vi "AlliGator Color Map Phasor in Original Image v3.vi"(7 "Image Color Scale Information":T2, 8 "Error In":errorcluster, 10 "Source Image Display":T1, 11 "AlliGator IV DVR in":refnum<data-value>) -> (0 "Error Out":errorcluster, 1 "# Overlay Pixels":i32, 2 "Source Image Display":T1, 3 "AlliGator IV DVR out":refnum<data-value>)   [LabVIEW 2021, in "AlliGator Phasor Plot Color Map.lvlib"]
doc: "Overlays a color-coded map on the Source Image based on the location of each pixel's phasor with respect to the user-defined <B>Color Map</B>, a polygon in the Phasor Plot, with one color associated with each vertex."
uses:
  AlliGator Phasor Plot Color Map.lvlib
  <vilib>/vision/Image Controls.llb/IMAQ Image.ctl
  Internal Variables/AlliGator Internal Variables v2.ctl
  Internal Variables/AlliGator Gate Image Set.ctl
  Files/AlliGator FLI Dataset Type.ctl
  Files/AlliGator Data Series Type.ctl
  Dual-Channel Datasets/AlliGator Dataset Channel.ctl
  Settings/AlliGator Gate Arithmetic.ctl
  Source Image/AlliGator Displayed Image.ctl
  Image/Named ROI Description.ctl
  Phasor Graph/AlliGator Decay Metadata v3.ctl
  Decay Analysis/Decay Preprocessing/AlliGator Decay Background Subtraction Info.ctl
  Decay Analysis/Decay Preprocessing/AlliGator Baseline Subtraction Method.ctl
  Graphs/XY Graph/XY Graph Plot Shift Parameters.ctl
  Graphs/XY Graph/XY Graph Plot Shift Method.ctl
  Decay Analysis/Decay Preprocessing/AlliGator Decay Extrapolation Parameters.ctl
  Phasor/Calibration Phasor (m, phi).ctl
  Phasor/Phasor Reference Series.ctl
  Phasor/Phasor Calibration Map v2.ctl
  Phasor/Phasor (g, s).ctl
  Phasor Graph/AlliGator Raw Phasor Plot Data v4.ctl
  Phasor/Phasor Standard Deviation Options.ctl
  Phasor Plot/AlliGator Phasor Multi-Harmonic Data.ctl
  Phasor/Phasor Harmonic Data.ctl
  Decay Fit Parameter Map/AlliGator Decay Fit Options & Parameters v2.ctl
  Fits/IRF(X)PSED/Decay Fit Options v2.ctl
  Fits/Decay Convolution/Decay Model.ctl
  Fits/Residual Type.ctl
  Fits/IRF(X)PSED/Fit Weights Type.ctl
  Fits/Non-linear Fitting Method v2.ctl
  Fits/Fit Calculation Method.ctl
  Fits/Non-linear Fitting Algorithm.ctl
  Decay Analysis/Decay Fit/AlliGator Decay Fit Parameter Constraints 2.ctl
  Fits/IRF(X)PSED/Decay Fit Parameters In List.ctl
  Fits/IRF(X)PSED/MLE Baseline Offset Type.ctl
  Decay Analysis/Decay Preprocessing/AlliGator Decay Preprocessing Parameters.ctl
  Fits/IRF(X)PSED/Decay Fit Parameters & Derived Quantities List v2.ctl
  Decay Fit Parameter Map/AlliGator Parameter Maps Data.ctl
  Image/Image Color Scale Information.ctl
  Settings/AlliGator Settings List.ctl
  Palette/Image Palette Information.ctl
  Image/Image Display Palette Type.ctl
  Globals, Variables, Constants/AlliGator Variables List.ctl
  Variant/Variant to Data/Variant to Boolean.vi
  <vilib>/Analysis/geometry.llb/Point in Polygon (Scalar).vi
  Image/Image Get Pixel Color.vi
  Image/Adjust Pixel Overlay Brightness.vi
  <vilib>/vision/NI_Vision_Development_Module.lvlib
  Error/Error.lvlib
  Image/Image.lvlib
  <vilib>/Analysis/NI_AAL_Geometry.lvlib
  Settings/AlliGator Settings.lvlib
  Variant/Variant to Data/Variant to Data.lvlib
  Time/Time.lvlib
  Utilities/Utilities.lvlib
  Globals, Variables, Constants/AlliGator Globals, Variables & Constants.lvlib
  Palette/Palette.lvlib
  Phasor/Phasor.lvlib
  Decay Analysis/Decay Preprocessing/AlliGator Decay Preprocessing.lvlib
  Graphs/XY Graph/XY Graph Add-Ons.lvlib
  Phasor Graph/AlliGator Phasor Graph.lvlib
  Files/AlliGator Files.lvlib
  Phasor Plot/AlliGator Phasor Plot.lvlib
  Source Image/AlliGator Source Image.lvlib
  Internal Variables/AlliGator Internal Variables.lvlib
  Fits/Fits.lvlib
  Decay Analysis/Decay Fit/AlliGator Decay Fit.lvlib
  Decay Fit Parameter Map/AlliGator Decay Fit Parameter Map.lvlib
  Dual-Channel Datasets/AlliGator Dual-Channel Datasets.lvlib
panel:
  out "Overlay Copy (s)":dbl
  out "Overlay Erase (s)":dbl
  out "Overlay Compute (s)":dbl
  # "see the AlliGator License on the block diagram (Ctrl+E or Window:Show Block Diagram)"
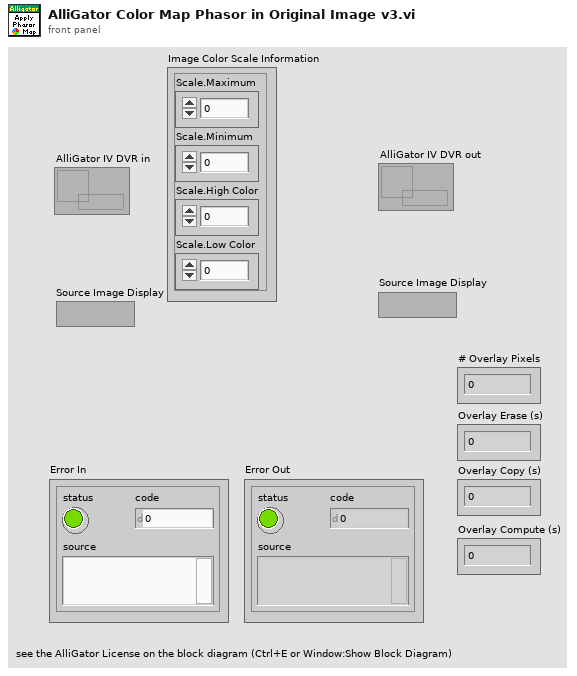
[diagram p1: front panel]
types:
  T1 = typedef "IMAQ Image.ctl" = refnum<image>
  T2 = typedef "Image.lvlib/Image Color Scale Information.ctl" = cluster{"Scale.Maximum":dbl, "Scale.Minimum":dbl, "Scale.High Color":u32, "Scale.Low Color":u32}
  T3 = typedef "AlliGator Settings.lvlib/AlliGator Settings List.ctl" = enum16{"GUI:Visible Settings Tab", "GUI:Last Run Version", "Source Image:Use Image Histogram for Contrast", "Source Image:Low Count Pixels Rejection Options", "Source Image:High Count Pixels Rejection Options", "Source Image:Use Image Brightness", "Source Image:Blend Overlay with Image Background", "Source Image:Use Fixed ROI Diameter", "Source Image:ROI Diameter", "Source Image:ROI Center Color", "Source Image:Peak Threshold", "Source Image:Intensity Threshold", "Source Image:Image Binning Options", "Source Image:Image Smoothing Options", "Source Image:Image Histogram Active", "Source Image:Invert Binary Mask", "Source Image:Hot Pixel Removal", "Source Image:Overlay Analyzed ROI Center", "Source Image:Auto-Adjust Contrast", "Source Image:Histogram Lower Percentile", "Source Image:Histogram Upper Percentile", "Source Image:Save Source Image", "Source Image:Scale Bar Options", "Source Image:Image Resolution (Pixel Size)", "Source Image:Flatfield Correction", "Source Image:Show Dead Left Columns Correction", "Source Image:Dead Left Columns Correction", "Source Image:Image Pre-Processing Operations Order", "Source Image:Overlay ROI Median", "Source Image:Median Overlay Color", "Data Information:Gate Width", "Data Information:Nanotime Gate Separation", "Data Information:Macrotime Gate Separation", "Data Information:Gate Step", "Data Information:# Gates", "Data Information:Gate Image Exposure", "Data Information:Gate Image Integration", "Data Information:Gates to Skip", "Data Information:Gates to Keep", "Data Information:Define Gates to", "Data Information:Channel Name", "Data Information:Available Channel Names", "Data Information:Channel Arithmetic", "Data Information:Background File Subtraction", "Data Information:Background File", "Data Information:Background Scaling Factor", "Data Information:Background Pile-up Correction", "Data Information:Background Pixel Well Capacity", "Data Information:Laser Period", "Data Information:SYNC Period", "Data Information:Pile-up Correction", "Data Information:Pixel Well Capacity", "Data Information:Dataset Scaling Factor", "Fluorescence Decay_Decay Pre-Processing:Reverse Gates", "Fluorescence Decay_Decay Pre-Processing:Verbose Decay Pre-Processing", "Fluorescence Decay_Decay Pre-Processing:Use Decay Pre-Processing", "Fluorescence Decay_Decay Pre-Processing:Background Subtraction", "Fluorescence Decay_Decay Pre-Processing:Background Definition Range", "Fluorescence Decay_Decay Pre-Processing:Baseline Subtraction Method", "Fluorescence Decay_Decay Pre-Processing:Decay Pre-Processing Operations Order", "Fluorescence Decay_Decay Pre-Processing:Smoothing Parameter", "Fluorescence Decay_Decay Pre-Processing:Shift Decay", "Fluorescence Decay_Decay Pre-Processing:Decay Shift Parameters", "Fluorescence Decay_Decay Pre-Processing:Fold Decay", "Fluorescence Decay_Decay Pre-Processing:# Folds", "Fluorescence Decay_Decay Pre-Processing:1-Normalize Decay", "Fluorescence Decay_Decay Pre-Processing:[0-1]-Normalize Decay", "Fluorescence Decay_Decay Pre-Processing:Smoothen Decay", "Fluorescence Decay_Decay Pre-Processing:Extrapolate Decay", "Fluorescence Decay_Decay Pre-Processing:Use Periodicity", "Fluorescence Decay_Decay Pre-Processing:Use Cursors", "Fluorescence Decay_Decay Pre-Processing:Tail Fraction", "Fluorescence Decay_Decay Pre-Processing:Head Fraction", "Fluorescence Decay_Decay Pre-Processing:Additional Points", "Fluorescence Decay_Decay Pre-Processing:Straighten Decay", "Fluorescence Decay_Decay Pre-Processing:Constant Background", "Fluorescence Decay_Decay Pre-Processing:Pixel-Normalize Decay", "Fluorescence Decay_Advanced Analysis:Extract IRF instead of Decay", "Fluorescence Decay_Advanced Analysis:IRF Extraction Options", "Fluorescence Decay_Advanced Analysis:IRF Optimization Options", "Fluorescence Decay_Advanced Analysis:Square Pulse Options", "Fluorescence Decay_Advanced Analysis:IRF Order", "Fluorescence Decay_Advanced Analysis:IRF Time Constants", "Fluorescence Decay_Advanced Analysis:Wavelet Analysis Options", "Fluorescence Decay_Advanced Analysis:Average Lifetime Options", "Fluorescence Decay_Fit Options:Fit Options", "Fluorescence Decay_Fit Options:Use Legacy Fitting Approach", "Fluorescence Decay_Fit Options:Use Data Information Laser Period", "Fluorescence Decay_Fit Parameters:Displayed Fit Parameters", "Fluorescence Decay_Fit Parameters:Fit Parameter Constraints", "Fluorescence Decay_Fit Parameters:Export Tabulated Results", "Fluorescence Decay_Fit Parameters:MLE Baseline Offset Type", "Fluorescence Decay_Fit Parameters:MLE Baseline Offset", "Fluorescence Decay_Fit Parameters:Guess Parameter Names", "Fluorescence Decay_Fit Parameters:Guess Parameter Values", "Fluorescence Decay_Fit Parameters:Guess Parameters Options", "Fluorescence Decay_Styles:Show Last Decay Only", "Fluorescence Decay_Styles:Decay Graph Color Array", "Fluorescence Decay:Decay Graph Active", "Fluorescence Decay Statistics:Min Peak Value", "Fluorescence Decay Statistics:Reject Low Decay Peak Pixels", "Fluorescence Decay Statistics:Reject High Decay Peak Pixels", "Fluorescence Decay Statistics:Max Peak Value", "Time Traces:Use File Timestamp", "Time Traces:Time Step", "Time Traces:Use Intensity Correction File", "Time Traces:Intensity Correction File", "Phasor Plot:Phasor Plot Smoothing Options", "Phasor Plot:Phasor Plot Size", "Phasor Plot:Phasor Plot Graphics Options", "Phasor Plot:Cumulative Phasor Plot", "Phasor Plot:Use Phasor Brightness", "Phasor Plot:Blend Overlay with Phasor Background", "Phasor Plot:Save Phasor Plot", "Phasor Plot:Show References", "Phasor Plot:Phasor Ratio Decay Range", "Phasor Plot:Exponential Fading", "Phasor Plot:Phasor Ratio Reference Colors", "Phasor Plot:Reference Radius", "Phasor Plot:Show Color Map Vertices", "Phasor Plot:Phasor Plot Active", "Phasor Plot:Phasor Ratio Color Map Type", "Phasor Plot:Phasor Ratio Color Map", "Phasor Plot:Phasor Ratio Display Range", "Phasor Plot:Selected Image ROI(s)", "Phasor Plot:All Image ROIs", "Phasor Plot:Selected Phasor Plot ROI(s)", "Phasor Plot:All Phasor Plot ROIs", "Phasor Plot:Phasor Ratio Color-Coded Quantity", "Phasor Plot:Store Phasor Harmonics", "Phasor Plot:Draw Reference Segment", "Phasor Plot:User-Defined Quantity", "Phasor Graph:Phasor Frequency", "Phasor Graph:Phasor Ratio Type", "Phasor Graph:Pixel-level Phasor Computation", "Phasor Graph:Save Phasor Graph", "Phasor Graph:Phasor Graph Active", "Phasor Graph:Phasor SDV Options", "Phasor Calibration:Use Backup Calibration if needed", "Phasor Graph:Define Shortest Lifetime as", "Phasor Calibration:Backup Calibration Type", "Phasor Calibration:Calibration Type", "Phasor Calibration:Calibration Lifetime", "Phasor Calibration:Calibration Map Algorithm", "Single-Exponential Phasor Locus (SEPL):Gate Parameters", "Single-Exponential Phasor Locus (SEPL):User-defined Gate", "Single-Exponential Phasor Locus (SEPL):User-defined IRF", "Single-Exponential Phasor Locus (SEPL):Phasor Parameters", "Single-Exponential Phasor Locus (SEPL):Decay & IRF Parameters", "Single-Exponential Phasor Locus (SEPL):Display Parameters", "Lifetime Analysis:Decay Analysis Parameters", "Lifetime Analysis:Lifetime Map Active", "Plugins:Python Settings", "Miscellaneous:Verbose Mode", "Miscellaneous:Beep after Script", "Miscellaneous:Saved Image File Format", "Miscellaneous:Exported Gate Image Settings", "Miscellaneous:Include Loading in Timing", "Miscellaneous:Verbose Settings Mode", "Miscellaneous:Histogram Options", "Miscellaneous:Beep on Error", "Miscellaneous:# Logical Processors Used", "Miscellaneous:ROI Description Max Characters", "Miscellaneous:Verbose Error Mode", "Miscellaneous:Transparent Mask Color"}
  T4 = typedef "Palette.lvlib/Image Palette Information.ctl" = cluster{"Palette Name [# Colors,int?,inv?]":string, "Palette Type":T5, "Palette Colors":u32[], "Interpolate?":bool}
  T5 = typedef "Image.lvlib/Image Display Palette Type.ctl" = u32
  T6 = typedef "AlliGator Globals, Variables & Constants.lvlib/AlliGator Variables List.ctl" = enum16{"---- GUI ----", "GUI:Initialization Status", "GUI:State Indicators Refnum", "GUI:Original AlliGator Menu Items", "GUI:Current Action Loop State", "GUI:Script in progress", "GUI:Playback", "GUI:Loop Playback", "GUI:Search ROI Used", "GUI:Search ROI", "Decay Graph Max Legend Size", "Intensity Graph Max Legend Size", "Decay Statistics Graph Max Legend Size", "Phasor Graph Max Legend Size", "Phasor Ratio Graph Max Legend Size", "Lifetime Graph Max Legend Size", "---- Files ----", "Files:Export Dataset Frames as Individual Files", "Files:Show Batch Export Help Balloons", "Files:Frames in Dataset", "Files:ptu File Frame Start Indices", "Files:Current Frame in Dataset", "Files:Current Frame Timestamp", "Files:Dataset Loaded", "Files:Dataset Metadata", "Files:Dataset Channel", "Files:Dataset Data Description", "Files:Background Dataset Metadata", "Files:Background Dataset Channel", "Files:Background Dataset Data Description", "Files:Background File Subtraction", "Files:Background File Path", "Files:Background File Pile-up Correction", "Files:Background File Pixel Well Capacity", "Files:Background File Scaling Factor", "Files:Current Dataset Load Settings", "Files:Dataset Path", "Files:ICCD-specific Information", "Files:Macrotime Gate Separation", "------ Python Plugins ------", "Python Plugins:Information", "Python Plugins:Python Session", "Python Plugins:Valid Python Session?", "---- Source Image ----", "Source Image:ROIs", "Source Image:Current ROI", "Source Image:ROI Event Refnum", "X_Source Image Display Range", "X_Source Image Palette Information", "X_Type of Displayed Image", "X_Time Gate Slider", "Source Image:Palette List", "Source Image:Scale", "Source Image:ROI Overlay Color", "Source Image:Overlay to Erase", "Source Image:Is Displayed Image Accumulated", "Source Image:White Light Image Modified", "Source Image:Mask Image Modified", "---- Image Profile Window ----", "Image Profile:Window Event Refnum", "Image Profile:IntensityType", "Image Profile:Intensity Average Type", "Image Profile:Intensity-weighted SDV", "Image Profile:Box Profile Type", "Image Profile:Window Open", "Image Profile:Plotted Fit Parameter", "------ Phasor Graph -------", "Phasor Graph:Show Line", "---- Phasor Plot ---", "Phasor Plot:Parameters Changed", "Phasor Plot:FLI Dataset Modified since last Calculation", "Phasor Harmonics Data", "Selected Phasor Harmonics", "Phasor Harmonic Manager Event Refnum", "Phasor Plot:ROIs", "Phasor Plot:Current ROI", "Phasor Plot:ROI Event Refnum", "Phasor Plot:Image Reference Points", "Phasor Plot:Computed", "Phasor Plot:Palette Information", "Phasor Plot:Palette List", "Phasor Plot:Phasor Ratio Palette Information", "Phasor Plot:Phasor Ratio Palette List", "Phasor Plot:Image Scale", "Phasor Plot:Image Overlay to Erase", "Phasor Plot:Image Elements to Update", "Phasor Plot:Current Calculation Parameters", "Phasor Plot:Current Calibration Options", "Phasor Plot:Reset Cumulated Phasor Plot", "Phasor Plot:Reference 1", "Phasor Plot:Lifetime Reference 1", "Phasor Plot:Reference 1 Frequency", "Phasor Plot:Reference 2", "Phasor Plot:Lifetime Reference 2", "Phasor Plot:Reference 2 Frequency", "---- Decay Analysis ----", "Number of Selected Decays to Fit", "LS Fit Results", "LAR Fit Results", "BS Fit Results", "Last Decay Max - Min", "Best Fit Parameters", "Best Fit Parameter Names", "Actual Size X", "Actual Size Y", "Binning X", "Binning Y", "Actual # Gates", "Dataset Number", "Gates to...", "Gates Skipped", "Gates to keep", "Gate Step", "Gate Separation", "Reversed Gates", "Pile-up Correction", "Pixel Well Capacity", "Background Subtracted", "Background Subtraction Method", "Background Definition Range", "Background File (deprecated)", "Number of Dataset Accumulated", "Array of Accumulated Dataset Paths", "Do Averaged Datasets", "Destination File Path", "Process Plot Target", "Use 1/D as Phasor Frequency", "---- Decay Fit Parameter Map -----", "Decay Fit Parameter Map:Palette Information", "Decay Fit Parameter Map:Palette List", "---- Parameter Map ----", "Parameter Map:Palette Information", "Parameter Map:Palette List", "------- Local Decay Window ---------", "Local Decay Graph Window:Event Refnum", "Local Decay Graph Window:Use normalized IRF for convolution", "----- Miscellaneous ----", "Misc:Skippable Dialog Windows Status"}
  T7 = typedef "AlliGator Internal Variables.lvlib/AlliGator Internal Variables v2.ctl" = cluster{"Displayed Image":T1, "White Light Image":T1, "Mask Image":T1, "ROI Mask Image":T1, "Current Dataset Images 1":T8, "Background Dataset Images 1":T8, "Current Dataset Images 2":T8, "Background Dataset Images 2":T8, "Current Dataset Arithmetic Images":T8, "Accumulated Dataset Images 1":T8, "Accumulated Dataset Images 2":T8, "Accumulated Dataset Arithmetic Images":T8, "Phasor Plot Image":T1, "Decay Fit Parameter Map Image":T1, "Parameter Map Image":T1, "Single Data Point Path":path, "White Light Image Path":path, "Mask Image Path":path, "Time-Series Folder":path, "[Time-Series Paths]":path[], "Current Dataset":i32, "Single Dataset Type":T9, "Current Folder":string, "AlliGator Data Series Type":T10, "# Datasets":i32, "Dual-Channel Dataset":bool, "Selected Channel Name":string, "Dataset Channel":T11, "Channel Arithmetic":T12, "Dual-Channel Background Dataset":bool, "Background Channel":T11, "Dual-Channel Accumulated Dataset":bool, "Start Time":dbl, "[Time-Series Timestamps]":dbl[], "[Intensity Corrections]":dbl[], "Time Series Script":bool, "Type of Displayed Image":T13, "Gate Image Slide":u16, "# Gates":i32, "ROIs":T14[], "ROI Decay":cluster{"t Array":dbl[], "I Array":dbl[]}, "Valid Decay":bool, "Decay  Metadata":T16, "Reference Decay Plot Name":string, "Reference Decay":cluster{"t Array":dbl[], "I Array":dbl[]}, "Decay Shift Plot":cluster{"Time Stamps":dbl[], "Decay Shifts":dbl[]}, "[Decays Max Values]":sgl[], "[Decays Min Values]":sgl[], "Calibration Phasor":T22, "Calibration Phasor Series":T23, "Phasor Calibration Map":T24, "Calibration Map MD5 Digest":string, "Last Raw Phasor":T25, "Last Calibrated Phasor":T25, "Last Calibrated Phasor SDV":T25, "Phasor Graph:Phasor Plot":cluster{"g Array":dbl[], "s Array":dbl[]}, "Phasor Graph:Phasor SDV Plot":cluster{"g Array":dbl[], "s Array":dbl[]}, "[Phasor Graph:Raw Phasor Plots]":T26[], "Phasor Plot locked to Ref 1":i32, "[Phasor Plot(s) locked to Ref 1]":i32[], "[Phasor Plot(s) locked to Ref 2]":i32[], "[Pixel Phasors]":T25[], "[[Sum Image]]":dbl[][], "[[CSG Phasors]]":csg[][], "[[Valid Pixel?]]":bool[][], "I/m/phi Dataset":cluster{"I/m/phi Dataset?":bool, "Base Frequency":dbl[unit], "Harmonic Orders":u8[]}, "Multi Phasor Plot Data":T28, "Decay Fit Options & Parameters":T30, "Fit Options: Decay Preprocessing Parameters":T41, "Fit Options: Reference Decay":cluster{"t Array":dbl[], "I Array":dbl[]}, "Is Full Image Parameters Map":bool, "Is Single-Pixels Parameters Map":bool, "NLSF Parameters Map X Resolution":i32, "NLSF Parameters Map Y Resolution":i32, "[Single Decay Fit Parameters]":dbl[], "Fit Model":T32, "[[Multiple Decays Fit Parameters]]":dbl[][], "[[Multiple Decays Fit Parameter SDVs]]":dbl[][], "[[IRFs]]":dbl[][], "IRF Array Time Axis":dbl[], "Decay Array Time Axis":dbl[], "[Decay Fit Parameter Names]":T42[], "[[Phasor Ratios]]":dbl[][], "[[Average Lifetimes]]":dbl[][], "Amplitude Weighted Average Lifetime":bool, "[Decay Sum]":dbl[], "[Map Set Names]":string[], "[Parameter Maps]":T43[], "[[User-defined Quantities]]":dbl[][], "User-defined Quantity":string}
  T8 = typedef "AlliGator Internal Variables.lvlib/AlliGator Gate Image Set.ctl" = cluster{"SGL Image Max":T1, "SGL Image Sum":T1, "SGL Gate Images":T1[], "SGL Image Min":T1}
  T9 = typedef "AlliGator Files.lvlib/AlliGator FLI Dataset Type.ctl" = enum16{"HDF5 FLI Dataset", "Gate Image Folder", ".sdt FLI Dataset (Becker & Hickl)", ".ptu FLI Dataset (PicoQuant)", "SS1 FLI Dataset", "SS2 FLI Dataset", "I/m/phi Dataset", ".bin FLI Dataset (PicoQuant Binned)", ".bin FLI Dataset (Piccolo Binned)"}
  T10 = typedef "AlliGator Files.lvlib/AlliGator Data Series Type.ctl" = enum16{"Not a Supported Series", "Gate Images Folder Series", "SwissSPAD 2 Dataset Series", "B&H FLI Dataset Series", "PicoQuant PTU FLI Dataset Series", "PicoQuant BIN FLI Dataset Series", "Piccolo hist BIN FLI Dataset Series", "HDF5 FLI Dataset Series"}
  T11 = typedef "AlliGator Dual-Channel Datasets.lvlib/AlliGator Dataset Channel.ctl" = enum16{"G2", "INT"}
  T12 = typedef "AlliGator Settings.lvlib/AlliGator Gate Arithmetic.ctl" = enum16{"None", "INT-G2", "G2/INT*<INT>", "(1 - G2/INT)*<INT>"}
  T13 = typedef "AlliGator Source Image.lvlib/AlliGator Displayed Image.ctl" = enum16{"Single Gate", "Sum of All Gates", "Max of All Gates", "Min of All Gates", "-", "White Ligth Image", "Mask Image"}
  T14 = typedef "Image.lvlib/Named ROI Description.ctl" = cluster{"ROI Descriptor":T15, "ROI Name":string, "Overlay Color":u32}
  T15 = typedef "ROI Descriptor" = cluster{"Global Rectangle":i32[], "Contours":cluster{"ID":enum32{"External", "Internal"}, "Type":u32, "Coordinates":i32[]}[]}
  T16 = typedef "AlliGator Phasor Graph.lvlib/AlliGator Decay Metadata v3.ctl" = cluster{"ROI Descriptor":T15, "ROI Center":cluster{"X":i32, "Y":i32}, "Decay Background Subtraction Info":T17, "Decay Reverted":bool, "Decay Smoothened":bool, "Decay Straightened":bool, "Fitted Tau (Decay Straightening)":dbl, "Decay Shift Parameters":T19, "Decay Shifted":bool, "Decay Extrapolated":bool, "Decay Extrapolation Parameters":T21, "Decay Normalized":bool, "Fold Decay":bool, "# Folds":u32}
  T17 = typedef "AlliGator Decay Preprocessing.lvlib/AlliGator Decay Background Subtraction Info.ctl" = cluster{"Laser Period":dbl[unit], "Gate Duration":dbl[unit], "Baseline Subtraction Method":T18, "Background Definition Range":cluster{"Min Gate":dbl[unit], "Max Gate":dbl[unit]}, "Total Intensity w/o Bkgd Subtraction":dbl, "Bkgd-subtracted Intensity (exp)":dbl, "# Data Points":i32, "Background/Gate":dbl, "Fitted Lifetime":dbl[unit], "Bkgd-subtracted Intensity (theo)":dbl}
  T18 = typedef "AlliGator Decay Preprocessing.lvlib/AlliGator Baseline Subtraction Method.ctl" = enum16{"Mean", "Min", "Square Gated Single-Exponential", "File", "Constant"}
  T19 = typedef "XY Graph Add-Ons.lvlib/XY Graph Plot Shift Parameters.ctl" = cluster{"Type":T20, "Shift":dbl[unit], "Threshold":dbl, "Rotate":bool}
  T20 = typedef "XY Graph Add-Ons.lvlib/XY Graph Plot Shift Method.ctl" = enum16{"Default", "CFD", "Threshold", "Cross-Correlation"}
  T21 = typedef "AlliGator Decay Preprocessing.lvlib/AlliGator Decay Extrapolation Parameters.ctl" = cluster{"Additional Points":u32, "Head Fraction":dbl, "Fitted Tau":dbl, "Use Periodicity":bool, "Use Cursors":bool, "Tail Fraction":dbl}
  T22 = typedef "Phasor.lvlib/Calibration Phasor (m, phi).ctl" = cluster{"m":dbl, "phi":dbl, "Phasor Frequency":dbl[unit], "Reference Lifetime":dbl[unit]}
  T23 = typedef "Phasor.lvlib/Phasor Reference Series.ctl" = cluster{"m Array":dbl[], "phi Array":dbl[], "Phasor Frequency":dbl[unit], "Calibration Lifetime":dbl[unit]}
  T24 = typedef "Phasor.lvlib/Phasor Calibration Map v2.ctl" = cluster{"Phasor Frequency":dbl[unit], "Calibration Lifetime":dbl[unit], "ROI Centers":cluster{"X":i32, "Y":i32}[], "ROI Descriptors":T15[], "Map Resolution X":i32, "Map Resolution Y":i32, "z Array":cdb[]}
  T25 = typedef "Phasor.lvlib/Phasor (g, s).ctl" = cluster{"g":dbl, "s":dbl}
  T26 = typedef "AlliGator Phasor Graph.lvlib/AlliGator Raw Phasor Plot Data v4.ctl" = cluster{"Phasor Plot Name":string, "Raw Phasor Plot":T25[], "Phasor Frequency":dbl[unit], "[Decay Metadata]":T16[], "Raw Phasor Plot SDV":T25[], "Phasor SDV Options":T27, "[Calibration Phasor]":T22[]}
  T27 = typedef "Phasor.lvlib/Phasor Standard Deviation Options.ctl" = cluster{"Compute Estimated SDV":bool, "# Replicas":u32, "Use Estimated Average Phasor":bool}
  T28 = typedef "AlliGator Phasor Plot.lvlib/AlliGator Phasor Multi-Harmonic Data.ctl" = cluster{"Base Frequency":dbl[unit], "# Harmonics":u8, "Harmonic Orders":u8[], "Phasor Plot Settings Checksum":u64, "Phasor Harmonic Data Array":T29[]}
  T29 = typedef "Phasor.lvlib/Phasor Harmonic Data.ctl" = cluster{"Phasor Harmonic Name":string, "Phasor Plot Settings Checksum":u64, "Phasor Frequency":dbl[unit], "Base Frequency":dbl[unit], "Harmonic Order":u8, "Phasor Plot Parameters":string, "Phasor Array [[CSG]]":csg[][], "Dataset File Path":path}
  T30 = typedef "AlliGator Decay Fit Parameter Map.lvlib/AlliGator Decay Fit Options & Parameters v2.ctl" = cluster{"SYNC Period":dbl[unit], "Fit Options":T31, "Fit Parameter Constraints":T38[], "MLE Baseline Offset":dbl, "MLE Baseline Offset Type":T40}
  T31 = typedef "Fits.lvlib/Decay Fit Options v2.ctl" = cluster{"Show Fit Residuals":bool, "Fit Model":T32, "Residual Type":T33, "Max Decay Percentile":dbl, "Min Decay Percentile":dbl, "Show Full Decay":bool, "Weights":T34, "Fitting Method":T35, "Compute Parameter Uncertainties":bool, "Periodic Boundaries":bool, "Model Calculation":T36, "Period":dbl[unit], "Termination Criteria":cluster{"Max Iterations":i32, "Max Function Calls":i32, "Max Time":dbl[unit], "Function Tolerance":dbl, "Parameter Tolerance":dbl, "Gradient Tolerance":dbl, "Min Lambda":dbl, "Max Lambda":dbl, "Initial Tick Count":u32}, "Offset Resolution":dbl[unit], "Use Local IRF":bool, "Fitting Algorithm":T37}
  T32 = typedef "Fits.lvlib/Decay Model.ctl" = enum16{"1-Exponential", "2-Exponentials"}
  T33 = typedef "Fits.lvlib/Residual Type.ctl" = enum16{"Standard", "Normalized", "Reduced"}
  T34 = typedef "Fits.lvlib/Fit Weights Type.ctl" = enum16{"Unweighted", "1/Variance", "Best of All"}
  T35 = typedef "Fits.lvlib/Non-linear Fitting Method v2.ctl" = enum16{"Least Square", "Least Absolute Residual", "Bisquare", "MLE", "-", "Best of All"}
  T36 = typedef "Fits.lvlib/Fit Calculation Method.ctl" = enum16{"Simulation", "Convolution", "Integration"}
  T37 = typedef "Fits.lvlib/Non-linear Fitting Algorithm.ctl" = enum16{"Levenberg-Marquardt", "Trust-Region Dogleg"}
  T38 = typedef "AlliGator Decay Fit.lvlib/AlliGator Decay Fit Parameter Constraints 2.ctl" = cluster{"Fit Parameter":T39, "Min Value":dbl, "Max Value":dbl, "Global":bool, "Used":bool}
  T39 = typedef "Fits.lvlib/Decay Fit Parameters In List.ctl" = enum16{"Offset", "Baseline", "A_1", "tau_1", "A_2", "tau_2"}
  T40 = typedef "Fits.lvlib/MLE Baseline Offset Type.ctl" = enum32{"Absolute", "Percentage"}
  T41 = typedef "AlliGator Decay Preprocessing.lvlib/AlliGator Decay Preprocessing Parameters.ctl" = cluster{"Background Subtraction":bool, "Straighten Decay":bool, "Reverse Gates":bool, "1-Normalized Decay":bool, "Smoothen Decay":bool, "Smoothing Parameter":dbl, "Shift Decay":bool, "Decay Shift Parameters":T19, "Extrapolate Decay":bool, "Additional Points":u32, "Head Fraction":dbl, "Pixel-Normalize Decay":bool, "Use Periodicity":bool, "Use Cursors":bool, "Tail Fraction":dbl, "Use Decay Pre-Processing":bool, "Fold Decay":bool, "# Folds":u32, "[0-1]-Normalized Decay":bool}
  T42 = typedef "Fits.lvlib/Decay Fit Parameters & Derived Quantities List v2.ctl" = enum16{"Offset", "Baseline", "A_1", "tau_1", "A_2", "tau_2", "<tau>_a", "f1_a", "f2_a", "<tau>_i", "f1_i", "f2_i", "-", "R^2", "Chi^2"}
  T43 = typedef "AlliGator Decay Fit Parameter Map.lvlib/AlliGator Parameter Maps Data.ctl" = cluster{"Map Set Name":string, "[Parameter Names]":string[], "[[Parameters]]":dbl[][], "[[Parameter SDVs]]":dbl[][], "Decay Array Time Axis":dbl[], "[[IRFs]]":dbl[][], "IRF Array Time Axis":dbl[]}
  T44 = cluster{"Red (or Hue) value":u8, "Green (or Sat) value":u8, "Blue (or Light or Val) value":u8}[]
  T45 = typedef "NI_AAL_Geometry.lvlib/Point in Polygon Position.ctl" = u16
  T46 = cluster{"Red (or Hue) value":u8, "Green (or Sat) value":u8, "Blue (or Light or Val) value":u8}
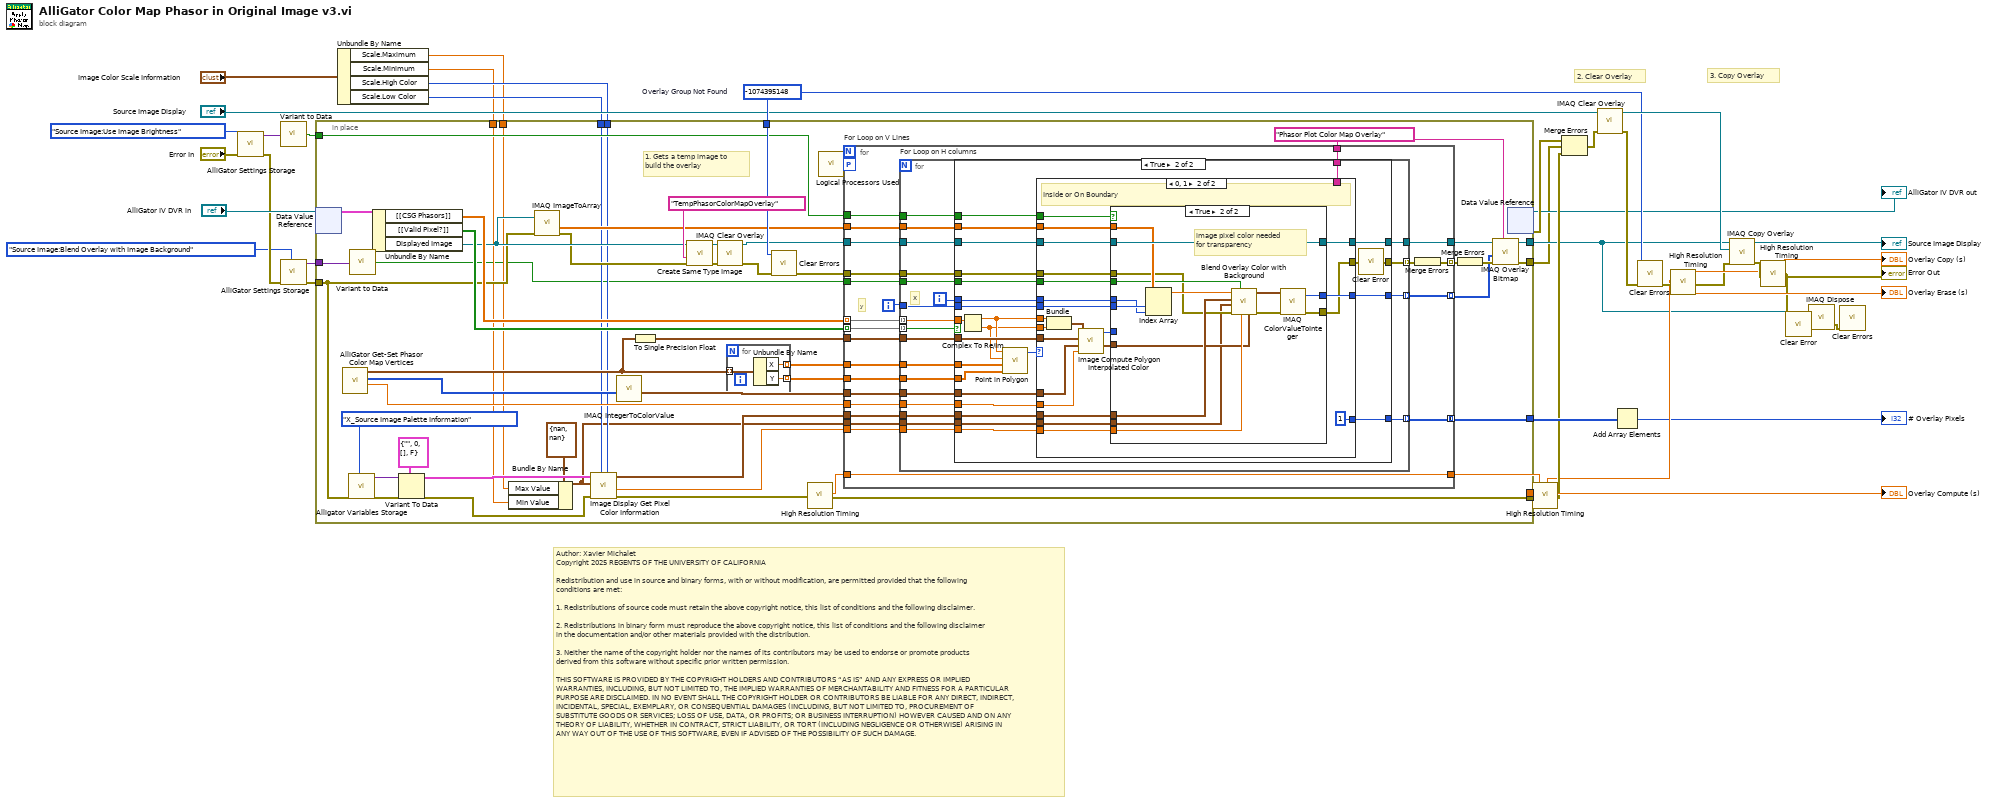
[diagram p0: block diagram]
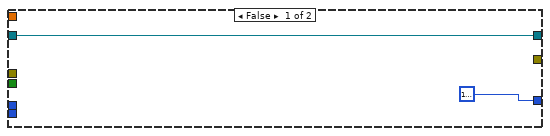
[diagram p2: hidden frame]
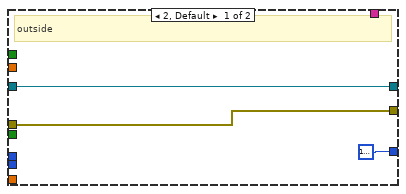
[diagram p3: hidden frame]
diagram:
  w34 = -1074395148  # Overlay Group Not Found
  # "Author: Xavier Michalet\nCopyright 2025 REGENTS OF THE UNIVERSITY OF CALIFORNIA\n\nRedistribution and use in source and binary forms, with or without modification, are permitted provided that the following conditions are met:\n\n1. Redistributions of source code must retain the above copyright notice, this list of conditions and the following disclaimer.\n\n2. Redistributions in binary form must reproduce the above copyright notice, this list of conditions and the following disclaimer in the documentation and/or other materials provided with the distribution.\n\n3. Neither the name of the copyright holder nor the names of its contributors may be used to endorse or promote products derived from this software without specific prior written permission.\n\nTHIS SOFTWARE IS PROVIDED BY THE COPYRIGHT HOLDERS AND CONTRIBUTORS “AS IS” AND ANY EXPRESS OR IMPLIED WARRANTIES, INCLUDING, BUT NOT LIMITED TO, THE IMPLIED WARRANTIES OF MERCHANTABILITY AND FITNESS FOR A PARTICULAR PURPOSE ARE DISCLAIMED. IN NO EVENT SHALL THE COPYRIGHT HOLDER OR CONTRIBUTORS BE LIABLE FOR ANY DIRECT, INDIRECT, INCIDENTAL, SPECIAL, EXEMPLARY, OR CONSEQUENTIAL DAMAGES (INCLUDING, BUT NOT LIMITED TO, PROCUREMENT OF SUBSTITUTE GOODS OR SERVICES; LOSS OF USE, DATA, OR PROFITS; OR BUSINESS INTERRUPTION) HOWEVER CAUSED AND ON ANY THEORY OF LIABILITY, WHETHER IN CONTRACT, STRICT LIABILITY, OR TORT (INCLUDING NEGLIGENCE OR OTHERWISE) ARISING IN ANY WAY OUT OF THE USE OF THIS SOFTWARE, EVEN IF ADVISED OF THE POSSIBILITY OF SUCH DAMAGE."
  # "3. Copy Overlay"
  # "2. Clear Overlay"
  n1 = call "AlliGator Settings Storage.vi"("AlliGator Settings List"=AlliGator_Settings_List."Source Image:Use Image Brightness", "Error In"="Error In") -> ("Error Out"=w4:errorcluster, "Variant Data out"=w36:variant)  [unwired: 8 in]
  n2 = call-poly "Variant to Data.vi"("Variant"=w36) -> ("Value"=w10:bool)  [unwired: 8 in]
  n3 = call "AlliGator Settings Storage.vi"("AlliGator Settings List"=AlliGator_Settings_List."Source Image:Blend Overlay with Image Background", "Error In"=w4) -> ("Error Out"=w3:errorcluster, "Variant Data out"=w1:variant)  [unwired: 8 in]
  n4 = Unbundle By Name("Image Color Scale Information") -> ("Scale.Maximum"=w6:dbl, "Scale.Minimum"=w7:dbl, "Scale.High Color"=w8:u32, "Scale.Low Color"=w9:u32)
  n5 = in-place {
    in-place-border: [w91] -> w40
    in-place-border: [w90] -> w18
    in-place-border: w3 -> [w64]
    in-place-border: w34 -> [w89]
    in-place-border: [w88] -> w33
    in-place-border: [w87] -> w32
    in-place-border: w10 -> [w60]
    in-place-border: w9 -> [w58]
    in-place-border: w8 -> [w57]
    in-place-border: w7 -> [w53]
    in-place-border: w6 -> [w52]
    in-place-border: [w49] -> w5
    in-place-border: w1 -> [w43]
    w75 = "Phasor Plot Color Map Overlay" ("Group")
    # "1. Gets a temp image to\nbuild the overlay"
    n6 = in-place-dvr #1("AlliGator IV DVR in") -> (w86:T7)  [unwired: 1 out]
    n7 = call "AlliGator Get-Set Phasor Color Map Vertices.vi"() -> ("Decay Range Exponent out"=w80:dbl, "Color Array out"=w83:u32[], "Vertices out"=w81:cluster{"X":dbl, "Y":dbl}[])  [unwired: 8 in, 1 out]
    n8 = call "Alligator Variables Storage.vi"("AlliGator Variable"=AlliGator_Variables_List."X_Source Image Palette Information" ("Alligator Variable"), "Error In"=w64) -> ("Error Out"=w63:errorcluster, "Data out"=w62:variant)  [unwired: 7 in, 1 out]
    n9 = call-poly "Variant to Data.vi"("Variant"=w43) -> ("Value"=w42:bool)  [unwired: 8 in]
    n10 = Unbundle By Name(w86) -> ("[[CSG Phasors]]"=w77:csg[][], "[[Valid Pixel?]]"=w76:bool[][], "Displayed Image"=w68:T1)
    n11 = Variant To Data(error in=w63, type=T4 {"Palette Name [# Colors,int?,inv?]"="", "Palette Type"=0, "Palette Colors"=[], "Interpolate?"=FALSE} ("Image Display Palette Information"), Variant=w62) -> (data=w59:T4, error out=w55:errorcluster)
    n12 = Bundle By Name(cluster=cluster{"Min Value":sgl, "Max Value":sgl} {"Min Value"=nan, "Max Value"=nan} ("Image Display Range"), "Max Value"=w52, "Min Value"=w53) -> (w41:cluster{"Min Value":sgl, "Max Value":sgl})
    n13 = call "IMAQ ImageToArray"("error in (no error)"=w64, "Image"=w68) -> ("Image Pixels (Float)"=w66:sgl[][], "error out"=w67:errorcluster)  [unwired: 2 in, 3 out]
    n14 = call "Image Display Get Pixel Color Information.vi"("Image High Color"=w57, "Image Low Color"=w58, "Error In"=w55, "Image Display Range"=w41, "Image Display Palette Information"=w59) -> ("Error Out"=w54:errorcluster, "Image Scale Factor (256 colors)"=w50:sgl, "1D Color Array"=w51:cluster{"Red":u8, "Green":u8, "Blue":u8}[])  [unwired: 3 in, 1 out]
    n15 = call "IMAQ IntegerToColorValue"("1D U32 array"=w83) -> ("1D Color value array"=w82:T44)  [unwired: 4 in, 3 out]
    n16 = To Single Precision Float(number=w81) -> (single precision float=w79:cluster{"X":sgl, "Y":sgl}[])
    n17 = call "Create Same Type Image.vi"("error in (no error)"=w67, "Name in"="TempPhasorColorMapOverlay", "Image Src"=w68) -> ("error out"=w72:errorcluster, "Image Dst"=w74:T1)  [unwired: 6 in, 1 out]
    n18 = call "IMAQ Clear Overlay"("error in (no error)"=w72, "Image"=w74) -> ("error out"=w71:errorcluster, "Image Out"=w73:T1)  [unwired: 8 in]
    n19 = for {
      tunnel: w81 -> [w209] mode=indexing
      tunnel: [w208] -> w85 mode=indexing
      tunnel: [w207] -> w84 mode=indexing
      n20 = Unbundle By Name(w209) -> ("X"=w208:dbl, "Y"=w207:dbl)
    }
    n21 = call <vilib>:"Clear Errors.vi"("error in (no error)"=w71, "specific error code to clear (0: all)"=w89) -> ("error out"=w70:errorcluster)  [unwired: 4 in, 1 out]
    n22 = call "High Resolution Timing.vi"("Error In"=w54) -> ("elapsed (relative) seconds"=w78:dbl, "Error Out"=w88:errorcluster)  [unwired: 16 in, 1 out]
    n23 = call "Logical Processors Used.vi"() -> ("# Logical Processor Used"=w48:i32)  [unwired: 6 in]
    n24 = for "For Loop on V Lines" {
      tunnel: w75 -> [w112]
      tunnel: w77 -> [w109] mode=indexing
      tunnel: w78 -> [w107]
      tunnel: [w107] -> w87
      tunnel: w85 -> [w106]
      tunnel: w84 -> [w105]
      tunnel: w82 -> [w104]
      tunnel: w79 -> [w103]
      tunnel: w80 -> [w102]
      tunnel: w60 -> [w101]
      tunnel: w76 -> [w100] mode=indexing
      tunnel: w73 -> [w113]
      tunnel: [w110] -> w47
      tunnel: w70 -> [w111]
      workers-P: w48 -> [_]
      tunnel: [w108] -> w91 mode=concatenating
      tunnel: w66 -> [w99]
      tunnel: w51 -> [w98]
      tunnel: w50 -> [w97]
      tunnel: [w96] -> w44 mode=indexing
      tunnel: [w94] -> w46 mode=indexing
      tunnel: w42 -> [w93]
      tunnel: w41 -> [w92]
      i -> [w114]
      # "y"
      n25 = for "For Loop on H columns" {
        tunnel: w114 -> [w124]
        tunnel: w112 -> [w135]
        tunnel: w109 -> [w129] mode=indexing
        tunnel: w106 -> [w131]
        tunnel: w105 -> [w130]
        tunnel: w104 -> [w128]
        tunnel: w103 -> [w127]
        tunnel: w102 -> [w126]
        tunnel: w101 -> [w125]
        tunnel: w100 -> [w122] mode=indexing
        tunnel: w113 -> [w136]
        tunnel: [w133] -> w110
        tunnel: w111 -> [w134]
        tunnel: [w132] -> w108 mode=indexing
        tunnel: w99 -> [w121]
        tunnel: w98 -> [w120]
        tunnel: w97 -> [w119]
        tunnel: [w118] -> w96 mode=indexing
        tunnel: [w117] -> w95 mode=indexing
        tunnel: w93 -> [w116]
        tunnel: w92 -> [w115]
        i -> [w123]
        # "x"
        n26 = case shown="True" w122 {
          tunnel: w136 -> [w138 w163]
          tunnel: w135 -> [_ w162]
          tunnel: w134 -> [_ w161]
          tunnel: [w138 w160] -> w133
          tunnel: [_ w159] -> w132
          tunnel: w131 -> [_ w158]
          tunnel: w130 -> [_ w157]
          tunnel: w129 -> [_ w156]
          tunnel: w128 -> [_ w155]
          tunnel: w127 -> [_ w154]
          tunnel: w126 -> [_ w151]
          tunnel: w125 -> [_ w150]
          tunnel: w124 -> [_ w148]
          tunnel: w123 -> [_ w149]
          tunnel: w121 -> [_ w147]
          tunnel: w120 -> [_ w146]
          tunnel: w119 -> [_ w145]
          tunnel: [u32 16777216 w144] -> w118
          tunnel: [_ w142] -> w117
          tunnel: w116 -> [_ w140]
          tunnel: w115 -> [_ w139]
          frame False {
          }
          frame True {
            n27 = Complex To Re/Im(x + iy=w156) -> (x=w153:sgl, y=w152:sgl)
            n28 = call-poly <vilib>:"Point in Polygon.vi"("Polygon Y"=w157, "Polygon X"=w158, "y"=w152, "x"=w153) -> ("position"=w141:T45)  [unwired: 6 in, 1 out]
            n29 = case shown="0, 1" w141 {
              tunnel: w163 -> [w165 w181]
              tunnel: w162 -> [_ _]
              tunnel: w161 -> [w166 w180]
              tunnel: [w166 w169] -> w143
              tunnel: [w165 w170] -> w160
              tunnel: [_ 1] -> w159
              tunnel: w155 -> [_ w188]
              tunnel: w154 -> [_ w187]
              tunnel: w153 -> [_ w186]
              tunnel: w152 -> [_ w185]
              tunnel: w151 -> [_ w183]
              tunnel: w150 -> [_ w182]
              tunnel: w149 -> [_ w179]
              tunnel: w148 -> [_ w178]
              tunnel: w147 -> [_ w174]
              tunnel: w146 -> [_ w173]
              tunnel: w145 -> [_ w172]
              tunnel: [u32 16777216 w171] -> w144
              tunnel: w140 -> [_ w168]
              tunnel: w139 -> [_ w167]
              frame 2, Default {
                # "outside"
              }
              frame 0, 1 {
                # "Inside or On Boundary"
                n30 = Bundle(w186, w185) -> (w184:cluster{sgl, sgl})  [unwired: 1 in]
                n31 = call "Image Compute Polygon Interpolated Color.vi"("Decay Range Exponent"=w183, "1D Color value array"=w188, "Vertices"=w187, "Pixel"=w184) -> ("Color Components"=w177:T46, "Color Value (U32)"=w176:u32)  [unwired: 6 in]
                n32 = case shown="True" w182 {
                  tunnel: w181 -> [w189 w204]
                  tunnel: w180 -> [w190 w195]
                  tunnel: w179 -> [_ w201]
                  tunnel: w178 -> [_ w202]
                  tunnel: w177 -> [_ w193]
                  tunnel: w176 -> [w191 _]
                  tunnel: [w191 w206] -> w171
                  tunnel: [w190 w205] -> w169
                  tunnel: [w189 w204] -> w170
                  tunnel: w174 -> [_ w203]
                  tunnel: w173 -> [_ w197]
                  tunnel: w172 -> [_ w194]
                  tunnel: w168 -> [_ w196]
                  tunnel: w167 -> [_ w192]
                  frame False {
                  }
                  frame True {
                    # "image pixel color needed\nfor transparency"
                    n33 = Index Array(array=w203, index (row)=w202, index (col)=w201) -> (element=w198:sgl)
                    n34 = call "Blend Overlay Color with Background.vi"("Overlay Color Value"=w193, "Image Scale Factor"=w194, "Blend Overlay with Background"=w196, "error in (no error)"=w195, "Image Display Range"=w192, "Image Color Array"=w197, "Pixel Value"=w198) -> ("error out"=w199:errorcluster, "Scaled/Blended Overlay Color Value"=w200:T46)  [unwired: 3 in]
                    n35 = call "IMAQ ColorValueToInteger"("error in (no error)"=w199, "Color Value"=w200) -> ("error out"=w205:errorcluster, "U32 value"=w206:u32)  [unwired: 3 in, 2 out]
                  }
                }
              }
            }
            n36 = call "Clear Error.vi"("Error In"=w143) -> ("no Error Out"=w142:errorcluster)  [unwired: 8 in]
          }
        }
      }
      n37 = Merge Errors(w95) -> (w94:errorcluster)
    }
    n38 = Merge Errors(w46) -> (w45:errorcluster)
    n39 = call "IMAQ Overlay Bitmap"("Group"=w75, "error in (no error)"=w45, "Bitmap"=w44, "Image"=w47) -> ("error out"=w49:errorcluster, "Image Out"=w90:T1)  [unwired: 6 in]
    n40 = in-place-dvr #1() -> (→"AlliGator IV DVR out":refnum<data-value>, w19:errorcluster)  [unwired: 1 in]
  }
  n41 = call "High Resolution Timing.vi"("relative seconds (NaN)"=w32, "Error In"=w33) -> ("relative seconds"=w28:dbl, "elapsed (relative) seconds"=→"Overlay Compute (s)":dbl, "Error Out"=w30:errorcluster)  [unwired: 15 in]
  n42 = Merge Errors(w19, w5, w30) -> (w20:errorcluster)
  n43 = call "IMAQ Clear Overlay"("error in (no error)"=w20, "Image"="Source Image Display") -> ("error out"=w35:errorcluster, "Image Out"=w39:T1)  [unwired: 8 in]
  n44 = Add Array Elements(numeric array=w40) -> (sum=→"# Overlay Pixels":i32)
  n45 = call <vilib>:"Clear Errors.vi"("error in (no error)"=w35, "specific error code to clear (0: all)"=w34) -> ("error out"=w29:errorcluster)  [unwired: 4 in, 1 out]
  n46 = call "High Resolution Timing.vi"("relative seconds (NaN)"=w28, "Error In"=w29) -> ("relative seconds"=w25:dbl, "elapsed (relative) seconds"=→"Overlay Erase (s)":dbl, "Error Out"=w23:errorcluster)  [unwired: 15 in]
  n47 = call "IMAQ Copy Overlay"("error in (no error)"=w23, "Image Dst"=w39, "Image Src"=w18) -> ("error out"=w26:errorcluster, "Image Dst Out"=→"Source Image Display":T1)  [unwired: 7 in]
  n48 = call "High Resolution Timing.vi"("relative seconds (NaN)"=w25, "Error In"=w26) -> ("elapsed (relative) seconds"=→"Overlay Copy (s)":dbl, "Error Out"=w12:errorcluster)  [unwired: 15 in, 1 out]
  "Error Out" <- w12
  n49 = call "Clear Error.vi"("Error In"=w12) -> ("no Error Out"=w14:errorcluster)  [unwired: 8 in]
  n50 = call "IMAQ Dispose"("Image"=w18, "error in (no error)"=w14) -> ("error out"=w17:errorcluster)  [unwired: 4 in]
  n51 = call <vilib>:"Clear Errors.vi"("error in (no error)"=w17) -> ()  [unwired: 5 in, 2 out]
